vi "Read_Electrical_Peripherals.vi"(8 "error in (no error)":errorcluster, 10 "Peripheral number":i32, 11 "Modbus master in":refnum<class "Modbus Master.lvclass">) -> (0 "error out":errorcluster, 2 "Variables":sgl[](array[numeric]), 3 "Modbus master out":refnum<class "Modbus Master.lvclass">)   [LabVIEW 2019]
uses:
  <vilib>/Modbus/master/Modbus Master.lvclass
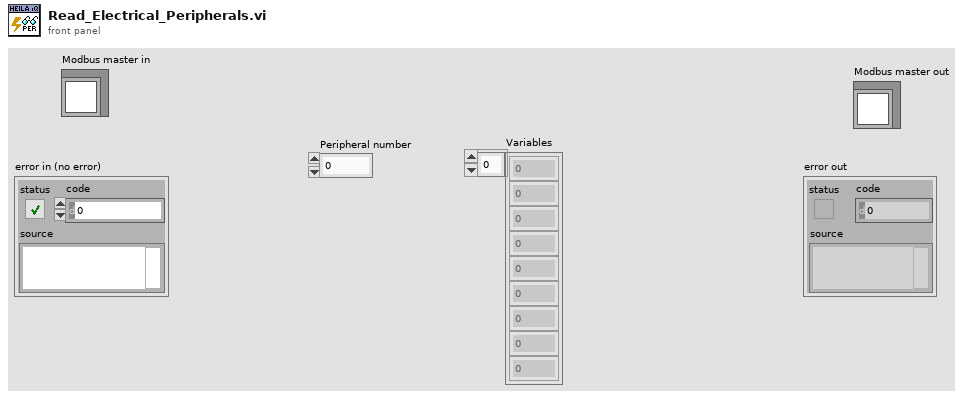
[diagram p1: front panel]
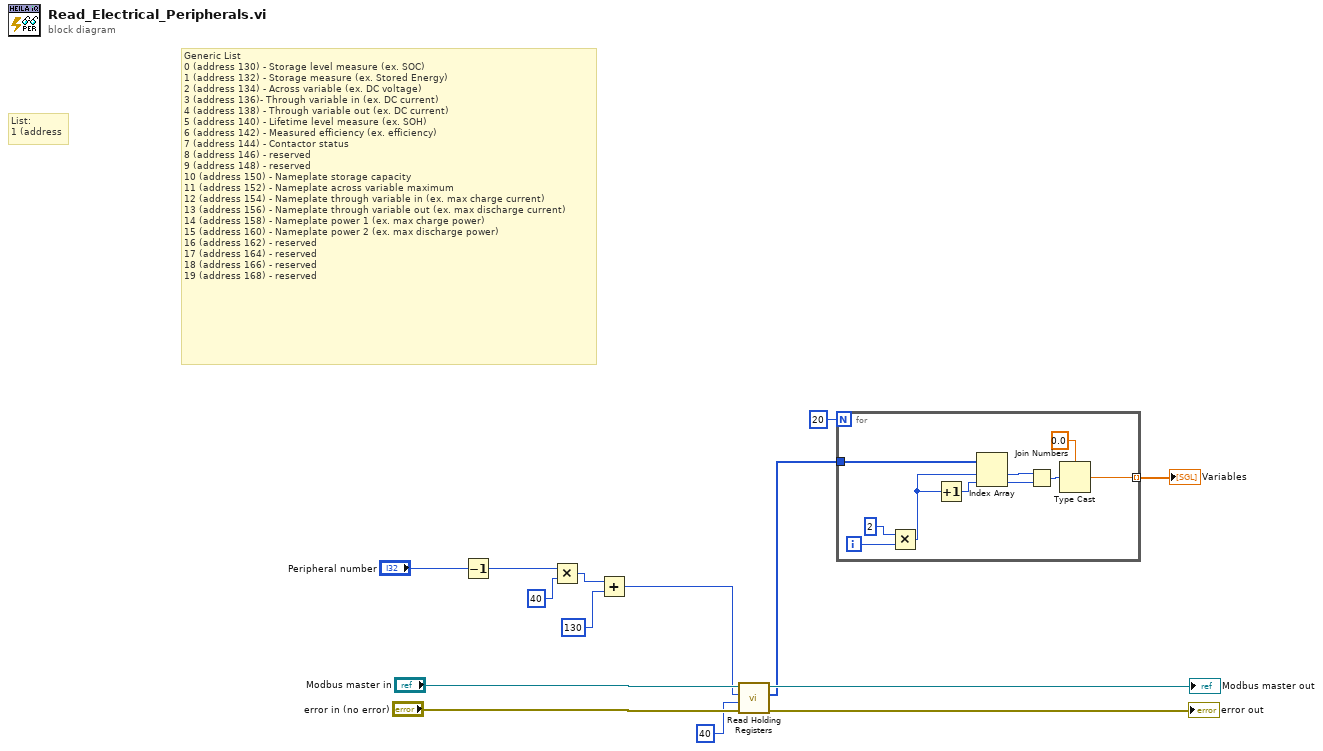
[diagram p0: block diagram]
diagram:
  # "Generic List\n0 (address 130) - Storage level measure (ex. SOC)\n1 (address 132) - Storage measure (ex. Stored Energy)\n2 (address 134) - Across variable (ex. DC voltage)\n3 (address 136)- Through variable in (ex. DC current)\n4 (address 138) - Through variable out (ex. DC current)\n5 (address 140) - Lifetime level measure (ex. SOH)\n6 (address 142) - Measured efficiency (ex. efficiency)\n7 (address 144) - Contactor status\n8 (address 146) - reserved\n9 (address 148) - reserved\n10 (address 150) - Nameplate storage capacity\n11 (address 152) - Nameplate across variable maximum\n12 (address 154) - Nameplate through variable in (ex. max charge current)\n13 (address 156) - Nameplate through variable out (ex. max discharge current)\n14 (address 158) - Nameplate power 1 (ex. max charge power)\n15 (address 160) - Nameplate power 2 (ex. max discharge power)\n16 (address 162) - reserved\n17 (address 164) - reserved\n18 (address 166) - reserved\n19 (address 168) - reserved"
  # "List:\n1 (address"
  n1 = Decrement(x="Peripheral number") -> (x-1=w4:i32)
  n2 = Multiply(x=w4, y=40) -> (x*y=w8:i32)
  n3 = Add(x=w8, y=u16 130 ("starting address")) -> (x+y=w6:i32)
  n4 = call-dynamic "Read Holding Registers.vi"("error in (no error)"="error in (no error)", "number of holding registers"=u16 40 ("starting address"), "starting address"=w6, "Modbus master in"="Modbus master in") -> ("error out"=→"error out":errorcluster, "register values"=w3:u16[], "Modbus master out"=→"Modbus master out":refnum<class "Modbus Master.lvclass">)  [unwired: 5 in]
  n5 = for {
    N: 20 -> [_]
    tunnel: w3 -> [w18]
    tunnel: [w15] -> w1 mode=indexing
    i -> [w16]
    n6 = Multiply(x=2, y=w16) -> (x*y=w17:i32)
    n7 = Increment(x=w17) -> (x+1=w19:i32)
    n8 = Index Array(array=w18, index #1=w17, index #2=w19) -> (element #1=w24:u16, element #2=w23:u16)
    n9 = Join Numbers(hi=w24, lo=w23) -> ((hi.lo)=w21:u32)
    n10 = Type Cast(type=sgl 0.0, x=w21) -> (*(type *) &x=w15:sgl)
  }
  "Variables" <- w1
